vi "Initialize Sim.vi"(8 "error in (no error)":errorcluster, 10 "Memory Size (32k)":i32=32768, 11 "Components (8)":i32=8) -> (0 "error out":errorcluster, 3 "FPGA Sim out":refnum<class "FPGA Sim.lvclass">)   [LabVIEW 2020, in "Unit Tests.lvlib" / "FPGA Sim.lvclass"]
uses:
  FPGA Sim.lvclass
  FPGA Sim.lvclass/FPGA Sim.ctl
  Dependencies/Virtual Memory Unit/Virtual Memory Unit.lvclass
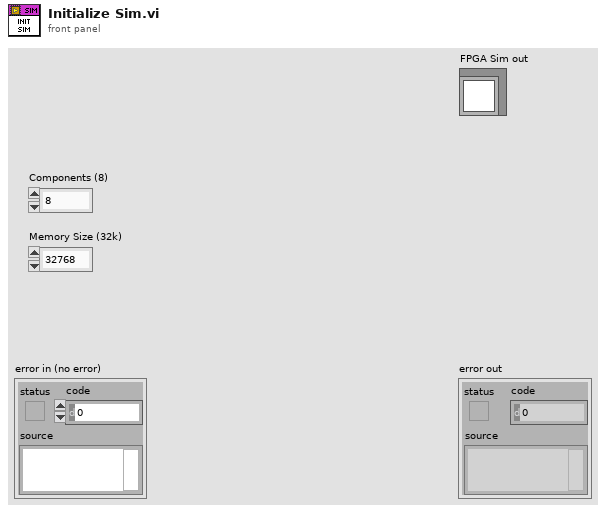
[diagram p1: front panel]
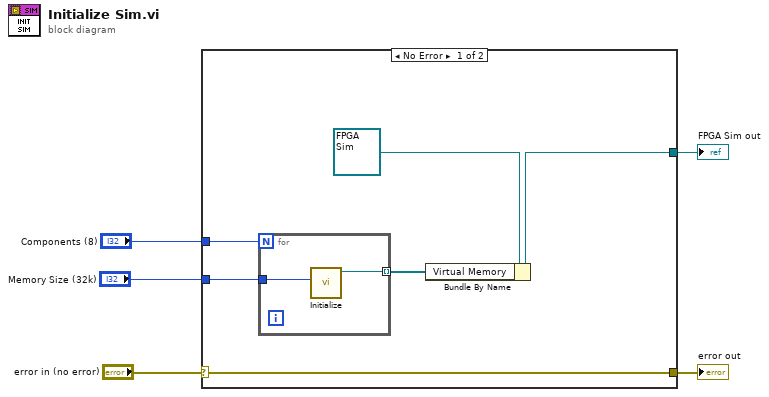
[diagram p0: block diagram]
diagram:
  n1 = case shown="No Error" "error in (no error)" {
    selector: "error in (no error)" -> [w11 w14]
    tunnel: [w11 w14] -> w4
    tunnel: [w7 _] -> w3
    tunnel: "Components (8)" -> [w10 _]
    tunnel: "Memory Size (32k)" -> [w9 _]
    frame No Error {
      n2 = for {
        N: w10 -> [_]
        tunnel: w9 -> [w13]
        tunnel: [w12] -> w6 mode=indexing
        n3 = call "Initialize.vi"("Memory Size"=w13) -> ("Virtual Memory Unit out"=w12:refnum<class "Virtual Memory Unit.lvclass">)  [unwired: 9 in, 1 out]
      }
      n4 = Bundle By Name(cluster=refnum<class "FPGA Sim.lvclass"> refnum ("FPGA Sim.lvclass"), "Virtual Memory"=w6) -> (w7:refnum<class "FPGA Sim.lvclass">)
    }
    frame Error {
    }
  }
  "error out" <- w4
  "FPGA Sim out" <- w3
